vi "Reports.Report Config - Read.vi"(7 "Config File":path, 8 "error in (no error)":errorcluster, 9 "Dialog":bool, 10 "Save Only":bool, 11 "Report Config In":T1[](array[typedef])) -> (0 "error out":errorcluster, 3 "Report Config Out":T1[](array[typedef]))   [LabVIEW 2018]
uses:
  Report.Report File Config Item.ctl
  Report.Report File Type.ctl
  <vilib>/KATE/Files/File Utils.lvlib
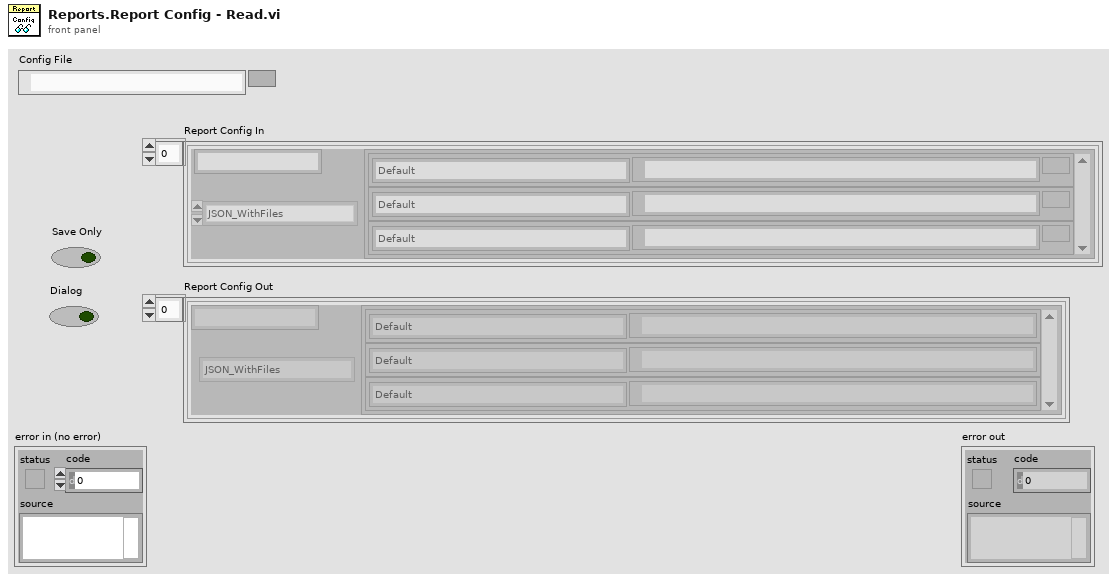
[diagram p1: front panel]
types:
  T1 = typedef "Report.Report File Config Item.ctl" = cluster{"Name":string, "Type":T2, "Seq_Dir":cluster{"Sequence":string, "Folder":path}[]}
  T2 = typedef "Report.Report File Type.ctl" = enum16{"CSV_WithConfigAndData", "CSV", "CSV_SummaryResult", "JSON", "JSON_WithFiles", "XLINK", "XLINK_ResultOnly", "SFC1", ""}
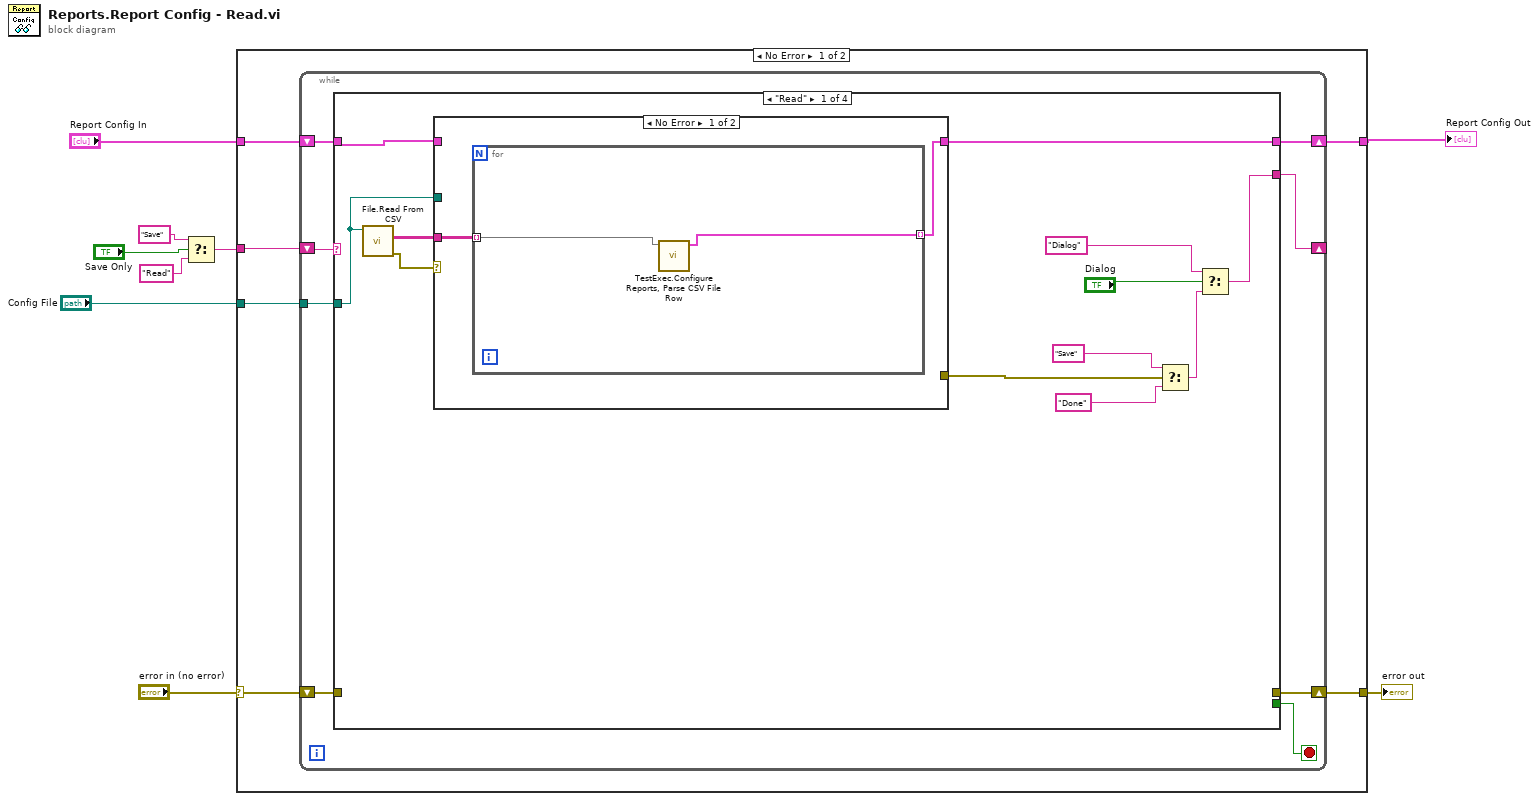
[diagram p0: block diagram]
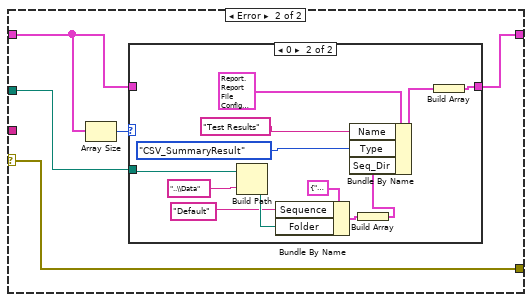
[diagram p2: hidden frame]
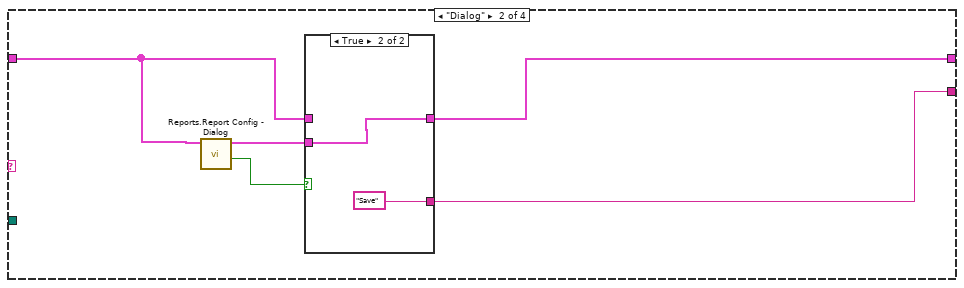
[diagram p4: hidden frame]
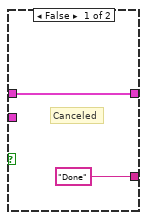
[diagram p5: hidden frame]
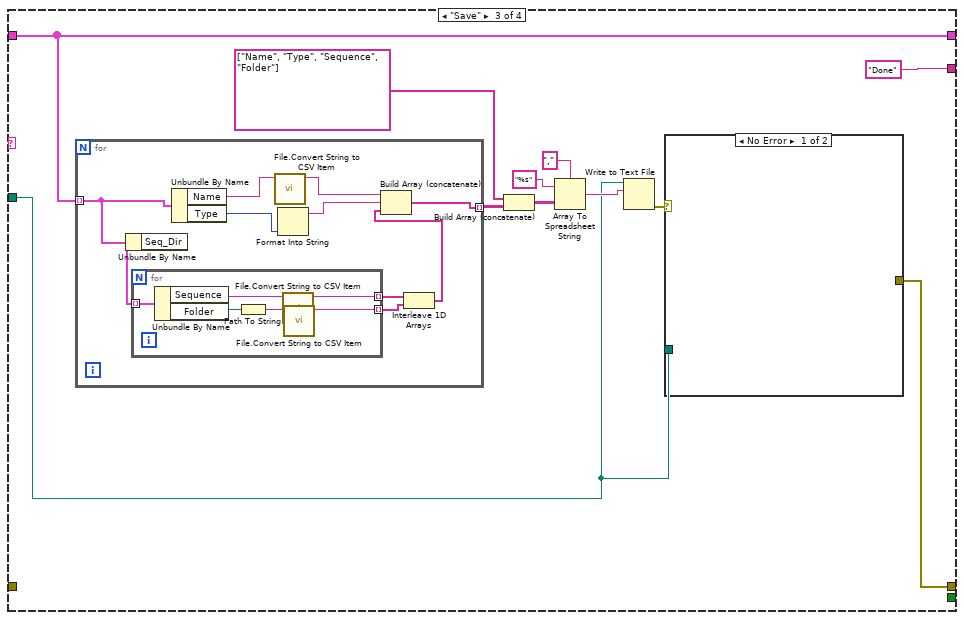
[diagram p6: hidden frame]
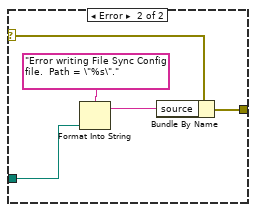
[diagram p7: hidden frame]
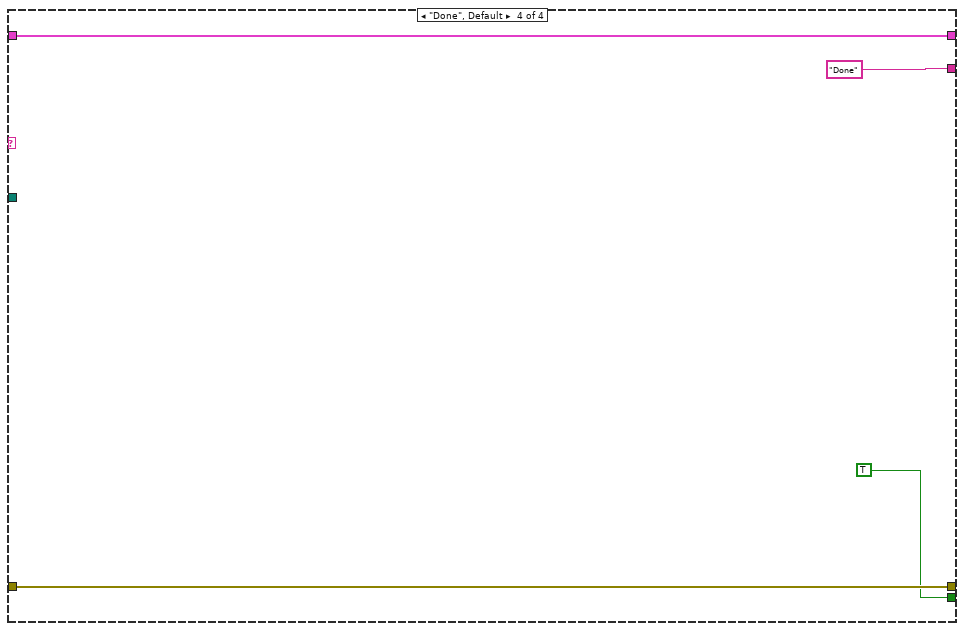
[diagram p8: hidden frame]
diagram:
  n1 = Select(t="Save", s="Save Only", f="Read") -> (s? t:f=w3:string)
  n2 = case shown="No Error" "error in (no error)" {
    selector: "error in (no error)" -> [w13 w104]
    tunnel: [w12 w104] -> w8
    tunnel: [w14 w103] -> w1
    tunnel: "Report Config In" -> [w10 w103]
    tunnel: "Config File" -> [w15 _]
    tunnel: w3 -> [w11 _]
    frame No Error {
      n3 = while {
        tunnel: w15 -> [w23]
        shift-right: [w21] -> w14
        shift-left: w10 -> [w22]
        shift-right: [w18] -> _
        shift-left: w11 -> [w19]
        shift-right: [w17] -> w12
        shift-left: w13 -> [w20]
        stop <- w16 stop-if-true
        n4 = case shown="\"Read\"" w19 {
          tunnel: w23 -> [w26 _ w69 _]
          tunnel: w22 -> [w25 w58 w67 w102]
          tunnel: [w31 w60 w67 w102] -> w21
          tunnel: w20 -> [_ _ _ w100]
          tunnel: [w32 w59 "Done" "Done"] -> w18
          tunnel: [_ _ w68 w100] -> w17
          tunnel: [_ _ _ TRUE] -> w16
          frame "Read" {
            n5 = call <vilib>:"File.Read From CSV.vi"("File"=w26) -> ("error out"=w30:errorcluster, "Data"=w35:string[][])  [unwired: 8 in, 1 out]
            n6 = case shown="No Error" w30 {
              selector: w30 -> [_ w44]
              tunnel: w35 -> [w37 _]
              tunnel: [w36 w41] -> w31
              tunnel: w25 -> [_ w42]
              tunnel: [_ w44] -> w24
              tunnel: w26 -> [_ w40]
              frame No Error {
                n7 = for {
                  tunnel: w37 -> [w39] mode=indexing
                  tunnel: [w38] -> w36 mode=indexing
                  n8 = call "TestExec.Configure Reports, Parse CSV File Row.vi"("Array"=w39) -> ("Report Config Item"=w38:T1)  [unwired: 10 in]
                }
              }
              frame Error {
                n9 = Array Size(array=w42) -> (size(s)=w43:i32)
                n10 = case shown="0" w43 {
                  tunnel: w42 -> [w45 _]
                  tunnel: [w45 w57] -> w41
                  tunnel: w40 -> [_ w52]
                  frame Default {
                  }
                  frame 0 {
                    n11 = Build Path(base path=w52, name or relative path="..\\Data") -> (appended path=w47:path)
                    n12 = Bundle By Name(cluster=cluster{"Sequence":string, "Folder":path} {"Sequence"="", "Folder"=path ""} ("Cluster"), "Sequence"="Default", "Folder"=w47) -> (w49:cluster{"Sequence":string, "Folder":path})
                    n13 = Build Array(w49) -> (w48:cluster{"Sequence":string, "Folder":path}[])
                    n14 = Bundle By Name(cluster=T1 {"Name"="", "Type"=enum."CSV_WithConfigAndData", "Seq_Dir"=[]} ("Report Config Item"), "Name"="Test Results", "Type"=Report.Report_File_Type."CSV_SummaryResult", "Seq_Dir"=w48) -> (w55:T1)
                    n15 = Build Array(w55) -> (w57:T1[])
                  }
                }
              }
            }
            n16 = Select(t="Save", s=w24, f="Done") -> (s? t:f=w27:string)
            n17 = Select(t="Dialog", s="Dialog", f=w27) -> (s? t:f=w32:string)
          }
          frame "Dialog" {
            n18 = call "Reports.Report Config - Dialog.vi"("Report Config"=w58) -> ("OK"=w62:bool, "Report Config Out"=w61:T1[])  [unwired: 9 in]
            n19 = case shown="True" w62 {
              tunnel: w61 -> [_ w65]
              tunnel: w58 -> [w64 _]
              tunnel: [w64 w65] -> w60
              tunnel: ["Done" "Save"] -> w59
              frame False {
                # "Canceled"
              }
              frame True {
              }
            }
          }
          frame "Save" {
            n20 = for {
              tunnel: w67 -> [w87] mode=indexing
              tunnel: [w92] -> w75 mode=indexing
              n21 = Unbundle By Name(w87) -> ("Seq_Dir"=w86:cluster{"Sequence":string, "Folder":path}[])
              n22 = for {
                tunnel: w86 -> [w97] mode=indexing
                tunnel: [w94] -> w85 mode=indexing
                tunnel: [w93] -> w84 mode=indexing
                n23 = Unbundle By Name(w97) -> ("Sequence"=w95:string, "Folder"=w96:path)
                n24 = Path To String(path=w96) -> (string=w98:string)
                n25 = call <vilib>:"File.Convert String to CSV Item.vi"("String"=w95) -> ("String Out"=w94:string)  [unwired: 10 in]
                n26 = call <vilib>:"File.Convert String to CSV Item.vi"("String"=w98) -> ("String Out"=w93:string)  [unwired: 10 in]
              }
              n27 = Unbundle By Name(w87) -> ("Name"=w91:string, "Type"=w89:T2)
              n28 = call <vilib>:"File.Convert String to CSV Item.vi"("String"=w91) -> ("String Out"=w90:string)  [unwired: 10 in]
              n29 = Format Into String(w89) -> (resulting string=w88:string)  [unwired: 3 in, 1 out]
              n30 = Interleave 1D Arrays(w85, w84) -> (w83:string[])
              n31 = Build Array (concatenate)(w90, w88, w83) -> (w92:string[])
            }
            n32 = Build Array (concatenate)(string[] ["Name", "Type", "Sequence", "Folder"], w75) -> (w74:string[][])
            n33 = Array To Spreadsheet String(delimiter (Tab)=",", array=w74, 3:"%s" ("format string")) -> (spreadsheet string=w71:string)
            n34 = Write to Text File(file (use dialog)=w69, text=w71) -> (error out=w70:errorcluster)  [unwired: 2 in, 2 out]
            n35 = case shown="No Error" w70 {
              selector: w70 -> [_ w82]
              tunnel: w69 -> [_ w79]
              tunnel: [_ w81] -> w68
              frame No Error {
              }
              frame Error {
                n36 = Format Into String(format string="Error writing File Sync Config file.  Path = \"%s\".", w79) -> (resulting string=w78:string)  [unwired: 2 in, 1 out]
                n37 = Bundle By Name(cluster=w82, "source"=w78) -> (w81:errorcluster)
              }
            }
          }
          frame "Done", Default {
          }
        }
      }
    }
    frame Error {
    }
  }
  "error out" <- w8
  "Report Config Out" <- w1
